vi "add PID to array.vi"(8 "error in":errorcluster, 10 "PID Element":T1={"Loop ID"="", "Tags"={"Setpoint"="", "Process Variable"="", "Output"=""}, "Gains"={"P"=1.0, "I"=0.01, "D"=0.0}, "Range"={"High"=100.0, "Low"=-100.0}}, 11 "operations table":T2) -> (0 "error out":errorcluster)   [LabVIEW 2014, in "Tagbus PID Module editor node.lvclass"]
uses:
  Tagbus PID Module editor node.lvclass
  PID array reference.ctl
  PID array element.ctl
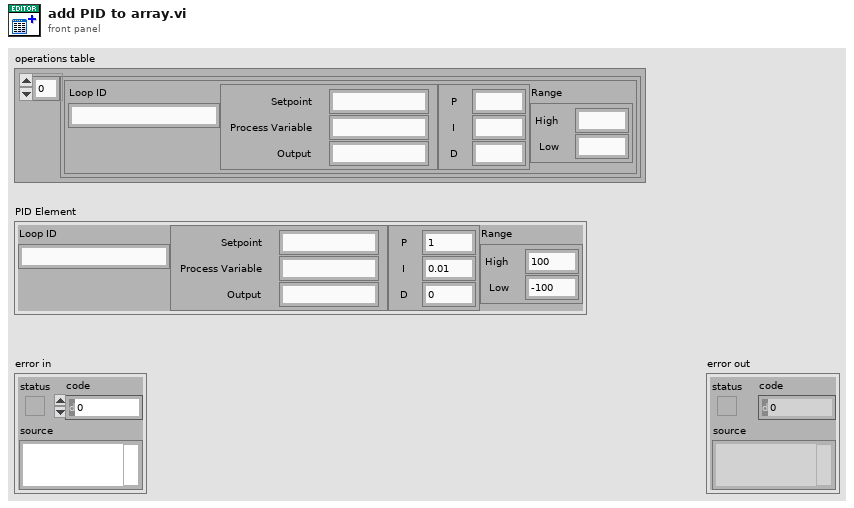
[diagram p1: front panel]
types:
  T1 = typedef "Tagbus PID Module editor node.lvclass/PID array element.ctl" = cluster{"Loop ID":string, "Tags":cluster{"Setpoint":string, "Process Variable":string, "Output":string}, "Gains":cluster{"P":dbl, "I":dbl, "D":dbl}, "Range":cluster{"High":dbl, "Low":dbl}}
  T2 = typedef "Tagbus PID Module editor node.lvclass/PID array reference.ctl" = refnum<vi>
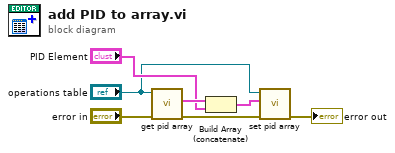
[diagram p0: block diagram]
diagram:
  n1 = call "get pid array.vi"("error in (no error)"="error in", "Array in"="operations table") -> ("error out"=w1:errorcluster, "Value"=w6:T1[])  [unwired: 7 in, 1 out]
  n2 = Build Array (concatenate)(w6, "PID Element") -> (w4:T1[])
  n3 = call "set pid array.vi"("error in (no error)"=w1, "Array"=w4, "Array in"="operations table") -> ("error out"=→"error out":errorcluster)  [unwired: 7 in, 1 out]
